vi "GetSignalSubset.vi"(10 "Selected Board":T1, 11 "Trigger Data Input":T4) -> (3 "Signal Subset":T2[](array[typedef]))   [LabVIEW 2016]
uses:
  Ctrl_Signal.ctl
  Ctrl_Signal_Map.ctl
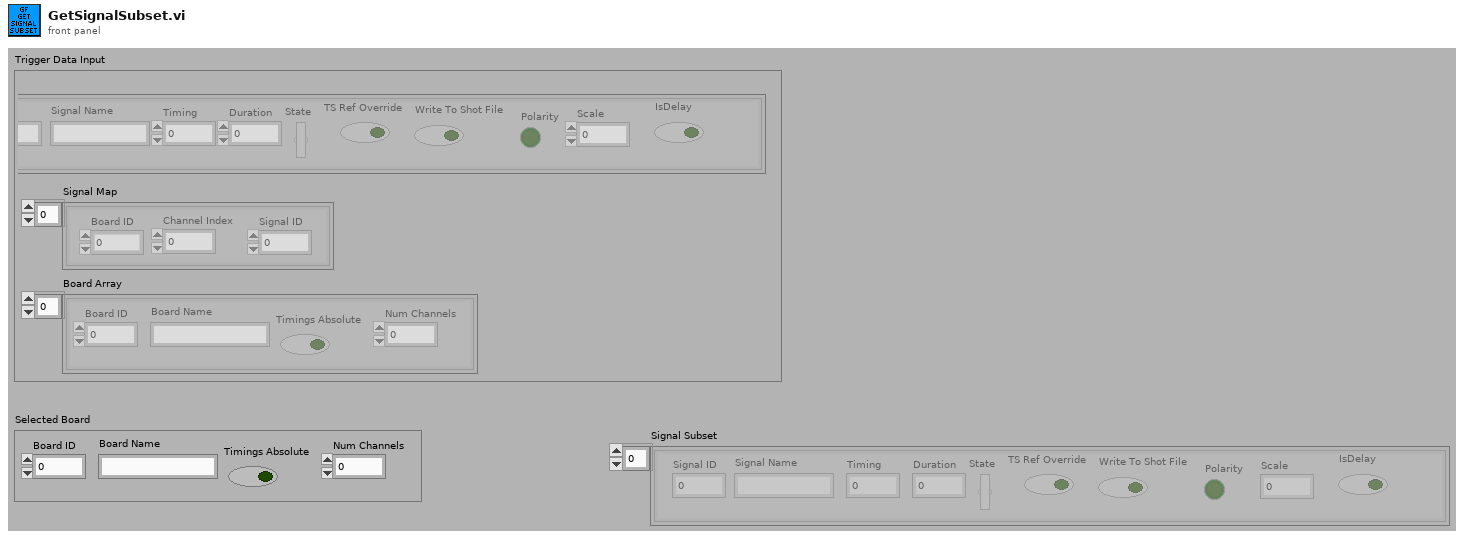
[diagram p1: front panel]
types:
  T1 = cluster{"Board ID":dbl, "Board Name":string, "Timings Absolute":bool, "Num Channels":dbl}
  T2 = typedef "Ctrl_Signal.ctl" = cluster{"Signal Name":string, "Timing":dbl, "Duration":dbl, "State":bool, "TS Ref Override":bool, "Write To Shot File":bool, "Polarity":bool, "Signal ID":dbl, "Scale":dbl, "IsDelay":bool}
  T3 = typedef "Ctrl_Signal_Map.ctl" = cluster{"Channel Index":dbl, "Board ID":dbl, "Signal ID":dbl}
  T4 = cluster{"Signal Array":T2[], "Signal Map":T3[], "Board Array":cluster{"Board ID":dbl, "Board Name":string, "Timings Absolute":bool, "Num Channels":dbl}[]}
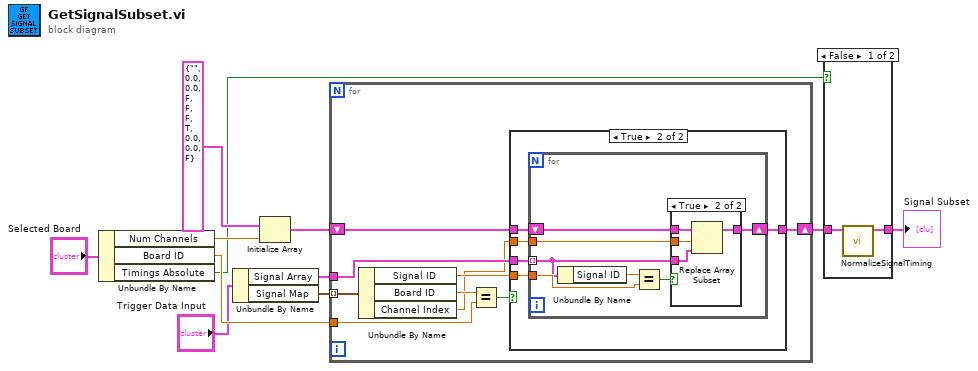
[diagram p0: block diagram]
diagram:
  n1 = Unbundle By Name("Selected Board") -> ("Num Channels"=w11:dbl, "Board ID"=w9:dbl, "Timings Absolute"=w1:bool)
  n2 = Unbundle By Name("Trigger Data Input") -> ("Signal Array"=w5:T2[], "Signal Map"=w6:T3[])
  n3 = Initialize Array(T2 {"Signal Name"="", "Timing"=0.0, "Duration"=0.0, "State"=FALSE, "TS Ref Override"=FALSE, "Write To Shot File"=FALSE, "Polarity"=TRUE, "Signal ID"=0.0, "Scale"=0.0, "IsDelay"=FALSE} ("Ctrl_Signal"), w11) -> (w8:T2[])
  n4 = for {
    tunnel: w6 -> [w20] mode=indexing
    tunnel: w5 -> [w19]
    tunnel: w9 -> [w17]
    shift-right: [w12] -> w2
    shift-left: w8 -> [w13]
    n5 = Unbundle By Name(w20) -> ("Signal ID"=w15:dbl, "Board ID"=w18:dbl, "Channel Index"=w14:dbl)
    n6 = Equal?(x=w18, y=w17) -> (x = y?=w16:bool)
    n7 = case shown="True" w16 {
      tunnel: w19 -> [_ w26]
      tunnel: w15 -> [_ w25]
      tunnel: w14 -> [_ w24]
      tunnel: w13 -> [w21 w23]
      tunnel: [w21 w22] -> w12
      frame False {
      }
      frame True {
        n8 = for {
          tunnel: w26 -> [w30] mode=indexing
          tunnel: w25 -> [w33]
          tunnel: w24 -> [w29]
          shift-right: [w27] -> w22
          shift-left: w23 -> [w28]
          n9 = Unbundle By Name(w30) -> ("Signal ID"=w32:dbl)
          n10 = Equal?(x=w32, y=w33) -> (x = y?=w31:bool)
          n11 = case shown="True" w31 {
            tunnel: w30 -> [_ w38]
            tunnel: w29 -> [_ w37]
            tunnel: w28 -> [w34 w36]
            tunnel: [w34 w35] -> w27
            frame False {
            }
            frame True {
              n12 = Replace Array Subset(array=w36, new element=w38, index=w37) -> (w35:T2[])
            }
          }
        }
      }
    }
  }
  n13 = case shown="False" w1 {
    tunnel: [w40 w41] -> w3
    tunnel: w2 -> [w39 w41]
    frame False {
      n14 = call "NormalizeSignalTiming.vi"("Input Signals"=w39) -> ("Aligned Signals"=w40:T2[])  [unwired: 10 in]
    }
    frame True {
    }
  }
  "Signal Subset" <- w3
